vi "GEN_Double Buttons ClueWindow.vi"(7 "Title Input":string="信息提示框", 8 "error in (no error)":errorcluster caption="错误输入（无错误）", 9 "Timeout":i32=-1, 10 "FP Action":T1(ring)=enum."Modal", 11 "Content Input":string="在此处添加对话框内容。\n\n提示：使用控件选板上系统类别中的控件，可令外观\n更为专业。\n\n请替换本文内容，或删除本标签。") -> (0 "error out":errorcluster caption="错误输出", 1 "Timeout?":bool, 3 "Cancelled?":bool caption="取消？")   [LabVIEW 2016]
doc: "该模板用于创建能够进行事件处理的对话框。"
panel:
  out "Content Display":string="在此处添加对话框内容。\n\n提示：使用控件选板上系统类别中的控件，可令外观\n更为专业。\n\n请替换本文内容，或删除本标签。"
  in  "Cancel":bool caption="取消"
  in  "OK":bool caption="确定"
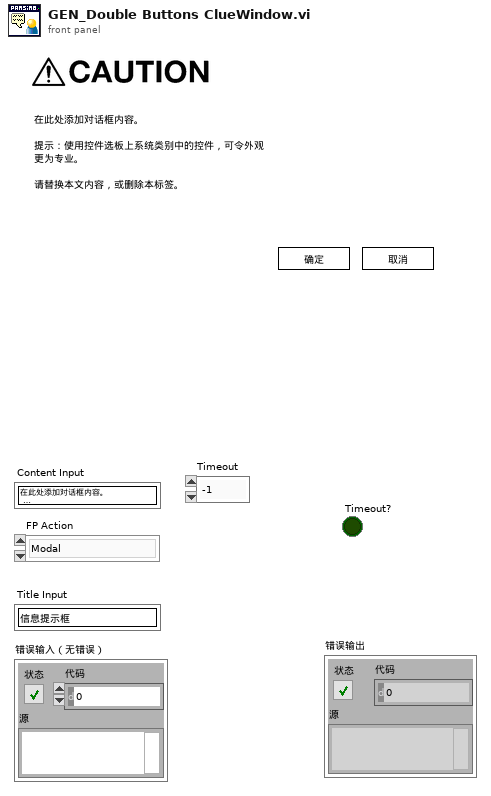
[diagram p1: front panel]
types:
  T1 = enum32{"Invalid", "Default", "Floating", "Floating/Auto-Hide", "Modal"}
  T2 = enum32{"Invalid", "Standard", "Closed", "Hidden", "Minimized", "Maximized"}
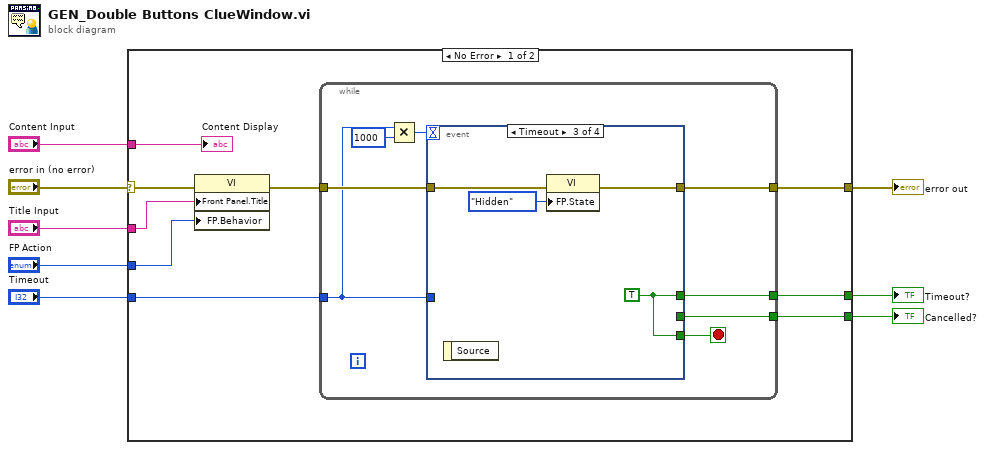
[diagram p0: block diagram]
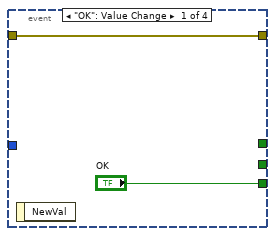
[diagram p2: hidden frame]
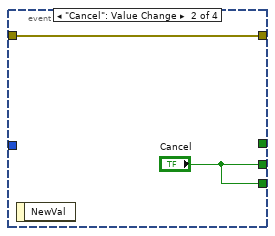
[diagram p3: hidden frame]
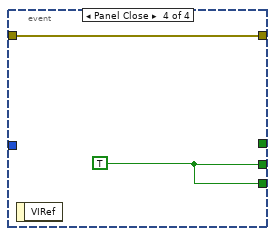
[diagram p4: hidden frame]
diagram:
  n1 = case shown="No Error" "error in (no error)" {
    selector: "error in (no error)" -> [w12 w36]
    tunnel: "Title Input" -> [w17 _]
    tunnel: [w16 w36] -> w7
    tunnel: "FP Action" -> [w14 _]
    tunnel: "Content Input" -> [w13 _]
    tunnel: "Timeout" -> [w11 _]
    tunnel: [w10 _] -> w2
    tunnel: [w9 _] -> w1
    frame No Error {
      n2 = property class="VI"(error in=w12, "Front Panel.Title"=w17, "FP.Behavior"=w14) -> (error out=w15:errorcluster)  [unwired: 1 in, 1 out]
      n3 = while {
        tunnel: [w24] -> w9
        tunnel: [w23] -> w16
        tunnel: w15 -> [w22]
        tunnel: w11 -> [w21]
        tunnel: [w18] -> w10
        stop <- w25 stop-if-true
        n4 = Multiply(x=w21, y=1000) -> (x*y=w19:i32)
        n5 = event shown="[2] Timeout" {
          selector: _ -> [_ _ _ _]
          dyn-events: _ -> [_ _ _ _]
          timeout: w19 -> [_ _ _ _]
          tunnel: ["OK" "Cancel" w33 w35] -> w25
          tunnel: [_ "Cancel" _ w35] -> w24
          tunnel: [w26 w28 w30 w34] -> w23
          tunnel: w22 -> [w26 w28 w31 w34]
          tunnel: w21 -> [_ _ _ _]
          tunnel: [_ _ w33 _] -> w18
          event "OK": Value Change {
            n6 = event-data() -> ()  [unwired: 1 in, 1 out]
          }
          event "Cancel": Value Change {
            n7 = event-data() -> ()  [unwired: 1 in, 1 out]
          }
          event Timeout {
            w33 = TRUE
            n8 = event-data() -> ()  [unwired: 1 in, 1 out]
            n9 = property class="VI"(error in=w31, "FP.State"=T2."Hidden" ("前面板窗口:状态")) -> (error out=w30:errorcluster)  [unwired: 1 in, 1 out]
          }
          event Panel Close {
            w35 = TRUE ("Stop?")
            n10 = event-data() -> ()  [unwired: 1 in, 1 out]
          }
        }
      }
      "Content Display" <- w13
    }
    frame Error {
    }
  }
  "error out" <- w7
  "Cancelled?" <- w1
  "Timeout?" <- w2
